vi "GetDescription.vi"(8 "Error In":errorcluster, 11 "reference in":refnum<class "ItalicDecorator.lvclass">) -> (0 "Error Out":errorcluster, 2 "Description":string, 3 "reference out":refnum<class "ItalicDecorator.lvclass">)   [LabVIEW 2024, in "ItalicDecorator.lvclass"]
uses:
  ItalicDecorator.lvclass
  IText/IText.lvclass
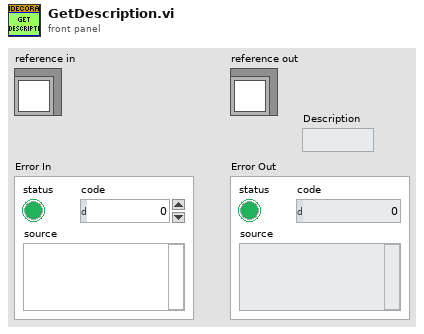
[diagram p1: front panel]
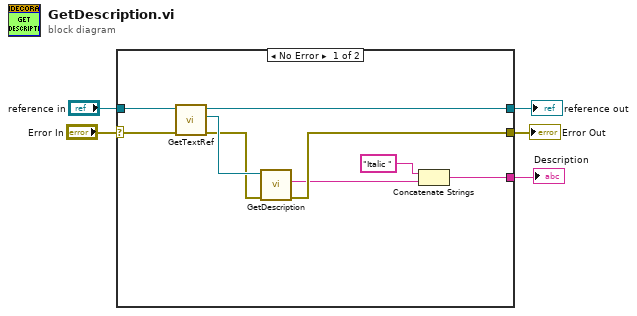
[diagram p0: block diagram]
diagram:
  n1 = case shown="No Error" "Error In" {
    selector: "Error In" -> [w14 w16]
    tunnel: [w9 w16] -> w4
    tunnel: [w12 w15] -> w2
    tunnel: "reference in" -> [w13 w15]
    tunnel: [w6 _] -> w1
    frame No Error {
      n2 = call-dynamic "GetTextRef.vi"("Error In"=w14, "reference in"=w13) -> ("Error Out"=w10:errorcluster, "TextRef"=w11:refnum<class "IText.lvclass">, "reference out"=w12:refnum<class "ItalicDecorator.lvclass">)  [unwired: 7 in]
      n3 = call-dynamic "GetDescription.vi"("Error In"=w10, "object in"=w11) -> ("Error Out"=w9:errorcluster, "Description"=w8:string)  [unwired: 7 in, 1 out]
      n4 = Concatenate Strings("Italic " ("string"), w8) -> (w6:string)
    }
    frame Error {
    }
  }
  "Error Out" <- w4
  "reference out" <- w2
  "Description" <- w1
